vi "Graphics-Boolean Matrix to Transparency Mask.vi"(11 "Mask In":bool[][](array[boolean])) -> (3 "Mask Out":u8[](array[numeric]))   [LabVIEW 2020]
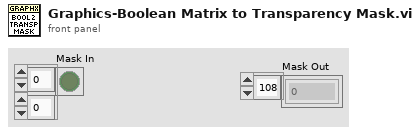
[diagram p1: front panel]
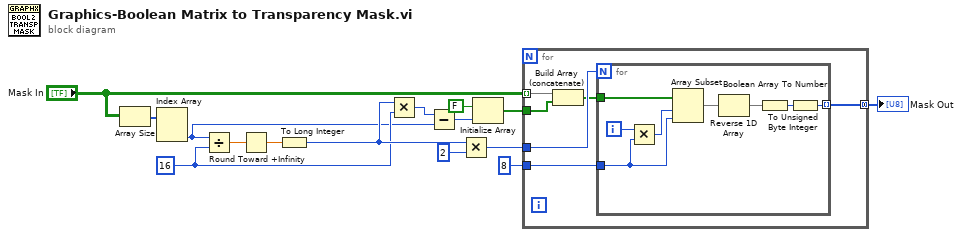
[diagram p0: block diagram]
diagram:
  w9 = 16 ("y")
  n1 = Array Size(array="Mask In") -> (size(s)=w14:i32[])
  n2 = Index Array(array=w14) -> (element #2=w7:i32)  [unwired: 2 in, 1 out]
  n3 = Divide(x=w7, y=w9) -> (x/y=w12:dbl)
  n4 = Round Toward +Infinity(x=w12) -> (ceil(x): smallest int >= x=w11:dbl)
  n5 = To Long Integer(number=w11) -> (32bit integer=w10:i32)
  n6 = Multiply(x=w10, y=w9) -> (x*y=w8:i32)
  n7 = Subtract(x=w8, y=w7) -> (x-y=w6:i32)
  n8 = Multiply(x=w10, y=2) -> (x*y=w3:i32)
  n9 = Initialize Array(FALSE, w6) -> (w4:bool[])
  n10 = for {
    tunnel: "Mask In" -> [w21] mode=indexing
    tunnel: [w20] -> w13 mode=concatenating
    tunnel: w3 -> [w19]
    tunnel: 8 -> [w18]
    tunnel: w4 -> [w16]
    n11 = Build Array (concatenate)(w21, w16) -> (w17:bool[])
    n12 = for {
      N: w19 -> [_]
      tunnel: w17 -> [w29]
      tunnel: [w26] -> w20 mode=indexing
      tunnel: w18 -> [w23]
      i -> [w25]
      n13 = Multiply(x=w25, y=w23) -> (x*y=w24:i32)
      n14 = Array Subset(array=w29, index=w24, length=w23) -> (w28:bool[])
      n15 = Reverse 1D Array(array=w28) -> (reversed array=w22:bool[])
      n16 = Boolean Array To Number(Boolean array=w22) -> (number=w27:u32)
      n17 = To Unsigned Byte Integer(number=w27) -> (unsigned 8bit integer=w26:u8)
    }
  }
  "Mask Out" <- w13
